vi "Comparison_Function.vi"(11 "Value of acceleration due to gravity":dbl) -> (3 "Within Specified Value?":bool)   [LabVIEW 2018]
doc: "This VI compares the experimental value of acceleration due to gravity and filters out the ones out of specified range.\n\nInputs:\nValue of acceleration due to gravity.\n\nOutputs:\nWithin Specified Value?."
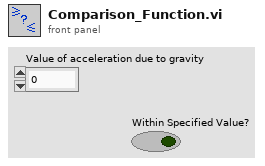
[diagram p1: front panel]
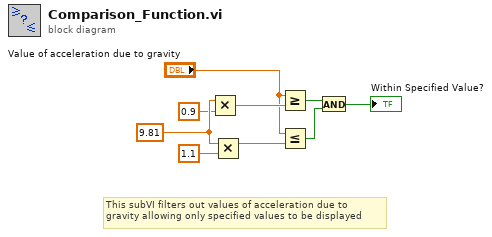
[diagram p0: block diagram]
diagram:
  w8 = 9.81 ("x")
  # "This subVI filters out values of acceleration due to\ngravity allowing only specified values to be displayed"
  n1 = Multiply(x=w8, y=0.9) -> (x*y=w5:dbl)
  n2 = Multiply(x=w8, y=1.1) -> (x*y=w7:dbl)
  n3 = Greater Or Equal?(x="Value of acceleration due to gravity", y=w5) -> (x >= y?=w1:bool)
  n4 = Less Or Equal?(x="Value of acceleration due to gravity", y=w7) -> (x <= y?=w2:bool)
  n5 = And(x=w1, y=w2) -> (x .and. y?=→"Within Specified Value?":bool)
